vi "Write SubComponent Scaled Data.vi"(5 "Component ID":u8, 7 "FPGA Interface":refnum<class "FPGA Interface.lvclass">, 8 "error in (no error)":errorcluster, 9 "Scaled Data":dbl[](array[numeric]), 10 "Parameters":string[](array[string]), 11 "1553 SubComponent in":refnum<class "1553 SubComponent.lvclass">) -> (0 "error out":errorcluster)   [LabVIEW 2020, in "BCI-1553 API.lvlib" / "1553 SubComponent.lvclass"]
doc: "Provides a means for taking in a parameter list and scaled value and writing it directly to a component in 1553 Session.\n\nThe parameter is cross-referenced to a memory address and the scaled data value is converted directly to a U16 before being written to the 1553 Session component in bulk."
uses:
  1553 SubComponent.lvclass
  Dependencies/FPGA Interface/FPGA Interface.lvclass
  1553 SubComponent.lvclass/1553 SubComponent.ctl
  Dependencies/Registry/Registry.lvclass/Registry.ctl
  Frames & Messages/TypeDefs/Parameter Table Data.ctl
  Frames & Messages/TypeDefs/Scaling Information.ctl
  Dependencies/Registry/Get Entry.vi
  BCI-1553 API.lvlib
  Dependencies/Registry/Registry.lvclass
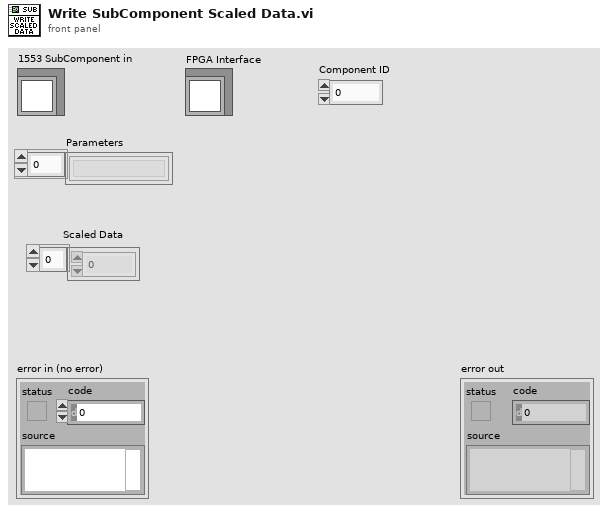
[diagram p1: front panel]
types:
  T1 = typedef "BCI-1553 API.lvlib/Parameter Table Data.ctl" = cluster{"Parameter Name":string, "Base Word":u16, "Address":u16, "Value":u64, "Mask":u16[], "Scaling Info":T2}
  T2 = typedef "BCI-1553 API.lvlib/Scaling Information.ctl" = cluster{"Bit Offset":i32, "Bit Count":i32, "LSB Resolution":dbl, "2's Complement":bool, "Big Endian":bool, "Sign Bit":bool}
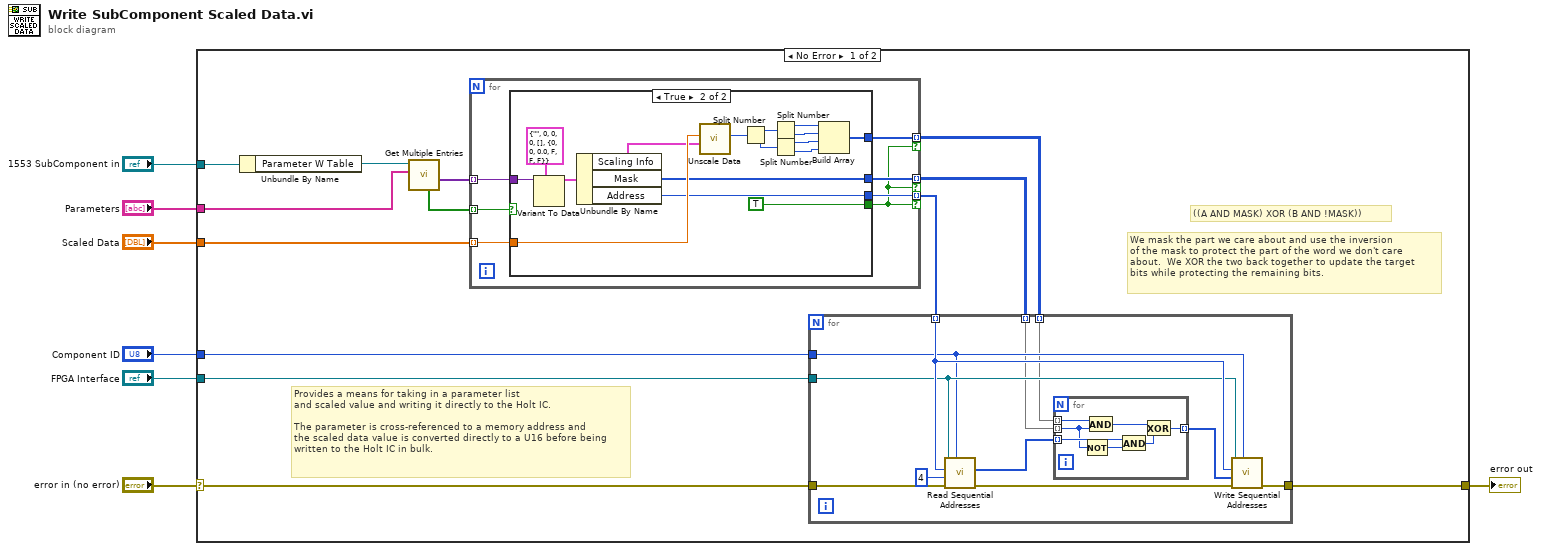
[diagram p0: block diagram]
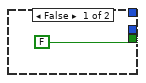
[diagram p2: hidden frame]
diagram:
  n1 = case shown="No Error" "error in (no error)" {
    selector: "error in (no error)" -> [w13 w63]
    tunnel: [w18 w63] -> w6
    tunnel: "1553 SubComponent in" -> [w20 _]
    tunnel: "Parameters" -> [w19 _]
    tunnel: "FPGA Interface" -> [w12 _]
    tunnel: "Component ID" -> [w17 _]
    tunnel: "Scaled Data" -> [w14 _]
    frame No Error {
      # "We mask the part we care about and use the inversion\nof the mask to protect the part of the word we don't care\nabout.  We XOR the two back together to update the target\nbits while protecting the remaining bits."
      # "((A AND MASK) XOR (B AND !MASK))"
      # "Provides a means for taking in a parameter list\nand scaled value and writing it directly to the Holt IC.\n\nThe parameter is cross-referenced to a memory address and\nthe scaled data value is converted directly to a U16 before being\nwritten to the Holt IC in bulk."
      n2 = Unbundle By Name(w20) -> ("Parameter W Table"=w8:refnum<class "Registry.lvclass">)
      n3 = call "Get Multiple Entries.vi"("Keys"=w19, "Registry in"=w8) -> ("Values"=w16:variant[], "Found?"=w15:bool[])  [unwired: 6 in, 2 out]
      n4 = for {
        tunnel: w16 -> [w43] mode=indexing
        tunnel: w15 -> [w45] mode=indexing
        tunnel: w14 -> [w44] mode=indexing
        tunnel: [w42] -> w9 mode=indexing if=w39
        tunnel: [w40] -> w11 mode=indexing if=w39
        tunnel: [w41] -> w10 mode=indexing if=w39
        n5 = case shown="True" w45 {
          tunnel: w44 -> [_ w60]
          tunnel: w43 -> [_ w62]
          tunnel: [_ w47] -> w42
          tunnel: [FALSE TRUE] -> w39
          tunnel: [_ w56] -> w41
          tunnel: [_ w55] -> w40
          frame False {
          }
          frame True {
            n6 = Variant To Data(type=T1 {"Parameter Name"="", "Base Word"=0, "Address"=0, "Value"=0, "Mask"=[], "Scaling Info"={"Bit Offset"=0, "Bit Count"=0, "LSB Resolution"=0.0, "2's Complement"=FALSE, "Big Endian"=FALSE, "Sign Bit"=FALSE}} ("Parameter Table Data"), Variant=w62) -> (data=w59:T1)  [unwired: 1 in, 1 out]
            n7 = Unbundle By Name(w59) -> ("Scaling Info"=w58:T2, "Mask"=w56:u16[], "Address"=w55:u16)
            n8 = call "Unscale Data.vi"("Scaling Info"=w58, "Scaled Value"=w60) -> ("Raw Value"=w48:u64)  [unwired: 8 in, 1 out]
            n9 = Split Number(x=w48) -> (hi(x)=w54:u32, lo(x)=w53:u32)
            n10 = Split Number(x=w54) -> (hi(x)=w52:u16, lo(x)=w51:u16)
            n11 = Split Number(x=w53) -> (hi(x)=w50:u16, lo(x)=w49:u16)
            n12 = Build Array(w52, w51, w50, w49) -> (w47:u16[])
          }
        }
      }
      n13 = for {
        tunnel: w17 -> [w26]
        tunnel: w12 -> [w27]
        tunnel: w13 -> [w29]
        tunnel: [w31] -> w18
        tunnel: w10 -> [w24] mode=indexing
        tunnel: w9 -> [w23] mode=indexing
        tunnel: w11 -> [w28] mode=indexing
        n14 = call-dynamic "Read Sequential Addresses.vi"("Target IC (1-8)"=w26, "error in (no error)"=w29, "Addresses to Read"=u16 4, "Starting Address"=w28, "FPGA Interface in"=w27) -> ("error out"=w30:errorcluster, "Data"=w25:u16[])  [unwired: 5 in]
        n15 = for {
          tunnel: w25 -> [w35] mode=indexing
          tunnel: w24 -> [w34] mode=indexing
          tunnel: w23 -> [w33] mode=indexing
          tunnel: [w32] -> w22 mode=indexing
          n16 = Not(x=w34) -> (.not. x?=w37:u16)
          n17 = And(x=w33, y=w34) -> (x .and. y?=w36:u16)
          n18 = And(x=w35, y=w37) -> (x .and. y?=w38:u16)
          n19 = Exclusive Or(1:w38, 2:w36) -> (0:w32:u16)
        }
        n20 = call-dynamic "Write Sequential Addresses.vi"("Target IC (1-8)"=w26, "error in (no error)"=w30, "Data"=w22, "Starting Address"=w28, "FPGA Interface in"=w27) -> ("error out"=w31:errorcluster)  [unwired: 6 in]
      }
    }
    frame Error {
    }
  }
  "error out" <- w6
